vi "CANrangeConfigurator.vi"(6 "timeoutSeconds":dbl=0.05, 8 "error in":errorcluster, 10 "DeviceConfiguration":T2={"Future Proof Configs"=FALSE, "CustomParamsCustomParam0"=0, "CustomParamsCustomParam1"=0, "ToFParamsUpdateMode"=0, "ToFParamsUpdateFrequency"=50.0, "ProximityParamsProximityThreshold"=0.4, "ProximityParamsProximityHysteresis"=0.01, "ProximityParamsMinSignalStrengthForValidMeasurement"=2500.0, "FovParamsFOVCenterX"=0.0, "FovParamsFOVCenterY"=0.0, "FovParamsFOVRangeX"=27.0, "FovParamsFOVRangeY"=27.0} {"ToFParamsUpdateMode" items=["ShortRange100Hz", "ShortRangeUserFreq", "LongRangeUserFreq"]}, 11 "DeviceReference":T1) -> (0 "error out":errorcluster)   [LabVIEW 2023]
uses:
  Users/test.DESKTOP-CORY/Documents/PhoenixProLabVIEWGeneration/CopyDown/DeviceReference.ctl
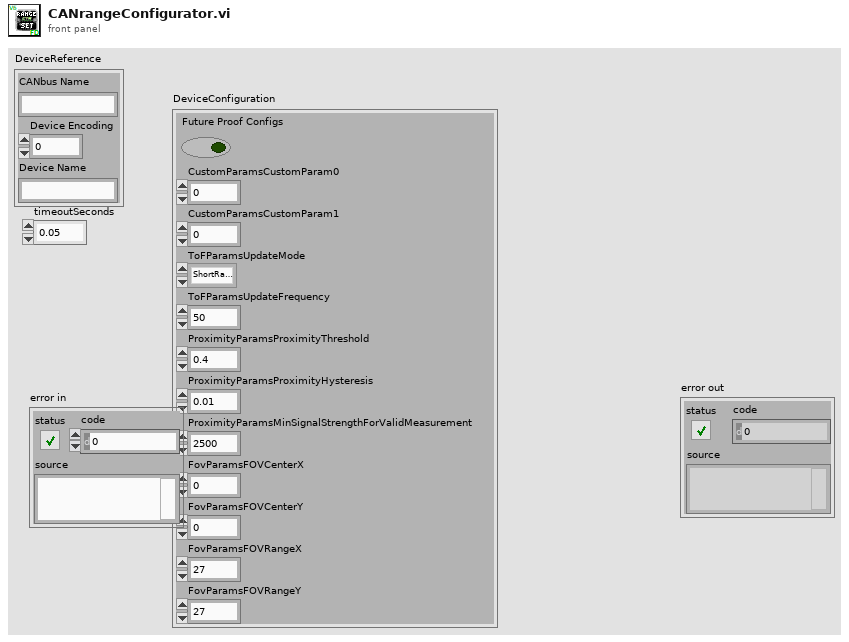
[diagram p1: front panel]
types:
  T1 = typedef "DeviceReference.ctl" = cluster{"CANbus Name":string, "Device Encoding":u32, "Device Name":string}
  T2 = cluster{"Future Proof Configs":bool, "CustomParamsCustomParam0":i16, "CustomParamsCustomParam1":i16, "ToFParamsUpdateMode":u16, "ToFParamsUpdateFrequency":dbl, "ProximityParamsProximityThreshold":dbl, "ProximityParamsProximityHysteresis":dbl, "ProximityParamsMinSignalStrengthForValidMeasurement":dbl, "FovParamsFOVCenterX":dbl, "FovParamsFOVCenterY":dbl, "FovParamsFOVRangeX":dbl, "FovParamsFOVRangeY":dbl}
  T3 = typedef "Type Descriptor Header__ogtk.ctl" = cluster{"length":u16, "private":u8, "type":T4, "# elements":u16}
  T4 = typedef "Type Descriptor Enumeration__ogtk.ctl" = enum8{"<Null>", "I8", "I16", "I32", "I64", "U8", "U16", "U32", "U64", "SGL", "DBL", "EXT", "CSG", "CDB", "CXT", "0x0F", "0x10", "0x11", "0x12", "0x13", "0x14", "Enum U8", "Enum U16", "Enum U32", "Enum U64", "SGL PQ", "DBL PQ", "EXT PQ", "CSG PQ", "CDB PQ", "CXT PQ", "0x1F", "0x20", "Boolean", "0x22", "0x23", "0x24", "0x25", "0x26", "0x27", "0x28", "0x29", "0x2A", "0x2B", "0x2C", "0x2D", "0x2E", "0x2F", "String", "0x31", "Path", "Pict", "0x34", "0x35", "0x36", "DAQ", "0x38", "0x39", "0x3A", "0x3B", "0x3C", "0x3D", "0x3E", "0x3F", "Array", "0x41", "0x42", "0x43", "0x44", "0x45", "0x46", "0x47", "0x48", "0x49", "0x4A", "0x4B", "0x4C", "0x4D", "0x4E", "0x4F", "Cluster", "0x51", "0x52", "Variant", "Waveform", "0x55", "0x56", "0x57", "0x58", "0x59", "0x5A", "0x5B", "0x5C", "0x5D", "0x5E", "Fixed Point", "0x60", "0x61", "0x62", "0x63", "0x64", "0x65", "0x66", "0x67", "0x68", "0x69", "0x6A", "0x6B", "0x6C", "0x6D", "0x6E", "0x6F", "Refnum", "0x71", "0x72", "Set Collection", "Map Collection"}
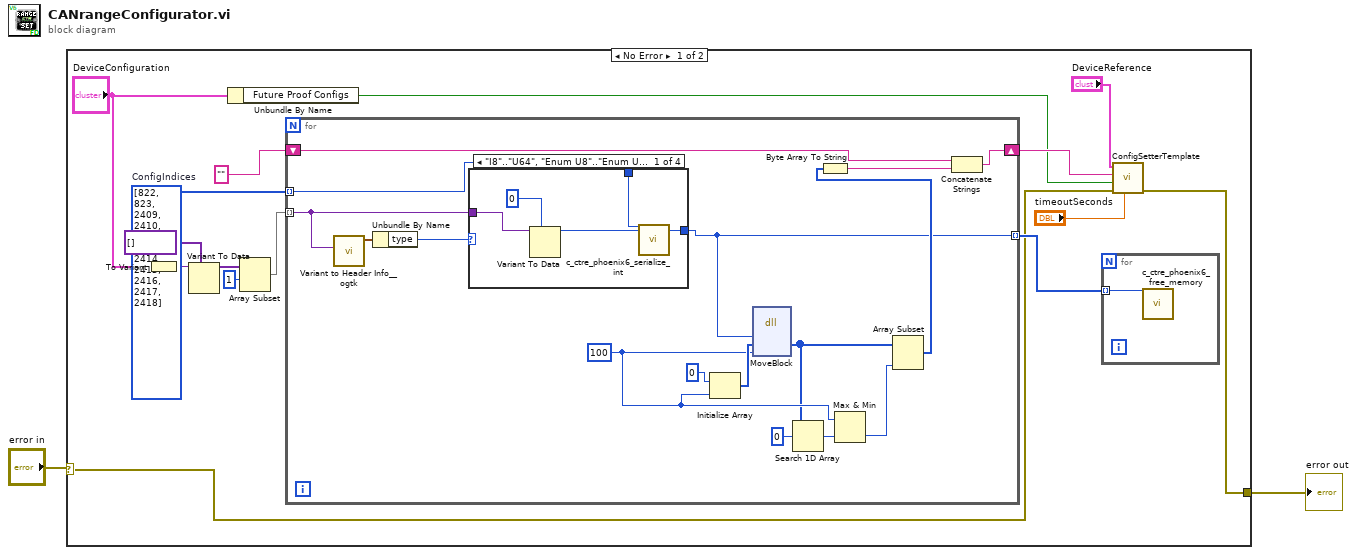
[diagram p0: block diagram]
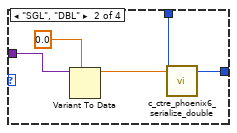
[diagram p2: hidden frame]
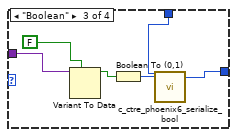
[diagram p3: hidden frame]
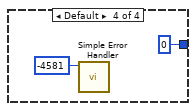
[diagram p4: hidden frame]
diagram:
  n1 = case shown="No Error" "error in" {
    selector: "error in" -> [w8 w53]
    tunnel: [w7 w53] -> w1
    frame No Error {
      w10 = i32[] [822, 823, 2409, 2410, 2412, 2413, 2414, 2415, 2416, 2417, 2418]  # ConfigIndices
      n2 = To Variant(anything="DeviceConfiguration") -> (Variant=w6:variant)
      n3 = Variant To Data(type=variant[] [], Variant=w6) -> (data=w3:variant[])  [unwired: 1 in, 1 out]
      n4 = Unbundle By Name("DeviceConfiguration") -> ("Future Proof Configs"=w9:bool)
      n5 = Array Subset(array=w3, index=1) -> (w12:variant[])  [unwired: 1 in]
      n6 = for {
        tunnel: w12 -> [w21] mode=indexing
        shift-right: [w32] -> w16
        shift-left: "" -> [w33]
        tunnel: [w18] -> w11 mode=indexing
        tunnel: w10 -> [w19] mode=indexing
        w25 = i64 100 ("size")
        n7 = call <userlib>:"Variant to Header Info__ogtk.vi"("Variant"=w21) -> ("Type Descriptor Header"=w22:T3)  [unwired: 3 in, 2 out]
        n8 = Unbundle By Name(w22) -> ("type"=w20:T4)
        n9 = case shown="\"I8\"..\"U64\", \"Enum U8\"..\"Enum U64\"" w20 {
          tunnel: w21 -> [w38 w43 w49 _]
          tunnel: w19 -> [w36 w40 w45 _]
          tunnel: [w34 w39 w44 u32 0 ("Numeric 4")] -> w18
          frame "I8".."U64", "Enum U8".."Enum U64" {
            n10 = Variant To Data(type=0, Variant=w38) -> (data=w35:i32)  [unwired: 1 in, 1 out]
            n11 = call <vilib>:"c_ctre_phoenix6_serialize_int.vi"("Numeric 2"=w36, "Numeric 3"=w35) -> ("Numeric 4"=w34:u32)  [unwired: 24 in, 1 out]
          }
          frame "SGL", "DBL" {
            n12 = Variant To Data(type=0.0, Variant=w43) -> (data=w41:dbl)  [unwired: 1 in, 1 out]
            n13 = call <vilib>:"c_ctre_phoenix6_serialize_double.vi"("Numeric 2"=w40, "Numeric 3"=w41) -> ("Numeric 4"=w39:u32)  [unwired: 24 in, 1 out]
          }
          frame "Boolean" {
            n14 = Variant To Data(type=FALSE, Variant=w49) -> (data=w47:bool)  [unwired: 1 in, 1 out]
            n15 = Boolean To (0,1)(Boolean=w47) -> (0, 1=w46:i16)
            n16 = call <vilib>:"c_ctre_phoenix6_serialize_bool.vi"("Numeric 2"=w45, "Numeric 3"=w46) -> ("Numeric 4"=w44:u32)  [unwired: 24 in, 1 out]
          }
          frame Default {
            n17 = call <vilib>:"Simple Error Handler.vi"("error code (no error:0)"=-4581) -> ()  [unwired: 4 in, 5 out]
          }
        }
        n18 = Initialize Array(u8 0 ("element"), w25) -> (w30:u8[])
        n19 = dll-call lib="LabVIEW" fn="MoveBlock"("ps"=w18, "pd"=w30, "size"=w25) -> ("pd"=w24:u8[])  [unwired: 6 in, 2 out]
        n20 = Search 1D Array(1D array=w24, element=u8 0) -> (index of element=w26:i32)  [unwired: 1 in]
        n21 = Max & Min(x=w25, y=w26) -> (min(x,y)=w23:i64)  [unwired: 1 out]
        n22 = Array Subset(array=w24, length=w23) -> (w28:u8[])  [unwired: 1 in]
        n23 = Byte Array To String(unsigned byte array=w28) -> (string=w31:string)
        n24 = Concatenate Strings(w33, w31) -> (w32:string)
      }
      n25 = for {
        tunnel: w11 -> [w52] mode=indexing
        n26 = call <vilib>:"c_ctre_phoenix6_free_memory.vi"("Numeric 3"=w52) -> ()  [unwired: 25 in, 2 out]
      }
      n27 = call <vilib>:"ConfigSetterTemplate.vi"("timeoutSeconds"="timeoutSeconds", "error in"=w8, "FutureProofConfigs"=w9, "Configs"=w16, "DeviceReference"="DeviceReference") -> ("error out"=w7:errorcluster)  [unwired: 6 in]
    }
    frame Error {
    }
  }
  "error out" <- w1
